vi "Execute Go Next Step.vi"(8 "error in (no error)":errorcluster, 11 "Chef Actor in":refnum<class "Chef Actor.lvclass">) -> (0 "error out":errorcluster, 3 "Chef Actor out":refnum<class "Chef Actor.lvclass">)   [LabVIEW 2024, in "Chef Actor.lvlib" / "Chef Actor.lvclass"]
uses:
  Chef Actor.lvclass
  Chef Actor.lvclass/Chef Actor.ctl
  Chef Actor Messages/Start Timer Msg/Start Timer Msg.lvclass
  Chef Actor Messages/Start Cooker Msg/Start Cooker Msg.lvclass
  <vilib>/ActorFramework/Actor/Actor.lvclass
  C:/Program Files/National Instruments/LabVIEW 2024/vi.lib/ActorFramework/Actor/Actor.lvclass
  G:/Leveling/LabVIEW/Learning/Actor Framework/chef/Chef Actor/Chef Actor.lvclass
  G:/Leveling/LabVIEW/Learning/Actor Framework/chef/Chef Actor Logic/Chef Actor Logic/Chef Actor Logic.lvclass
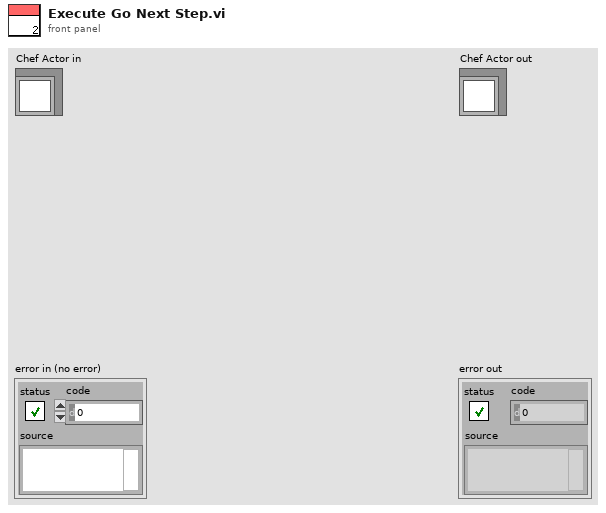
[diagram p1: front panel]
types:
  T1 = typedef "Step.ctl" = cluster{"Fire":dbl, "Duration":dbl}
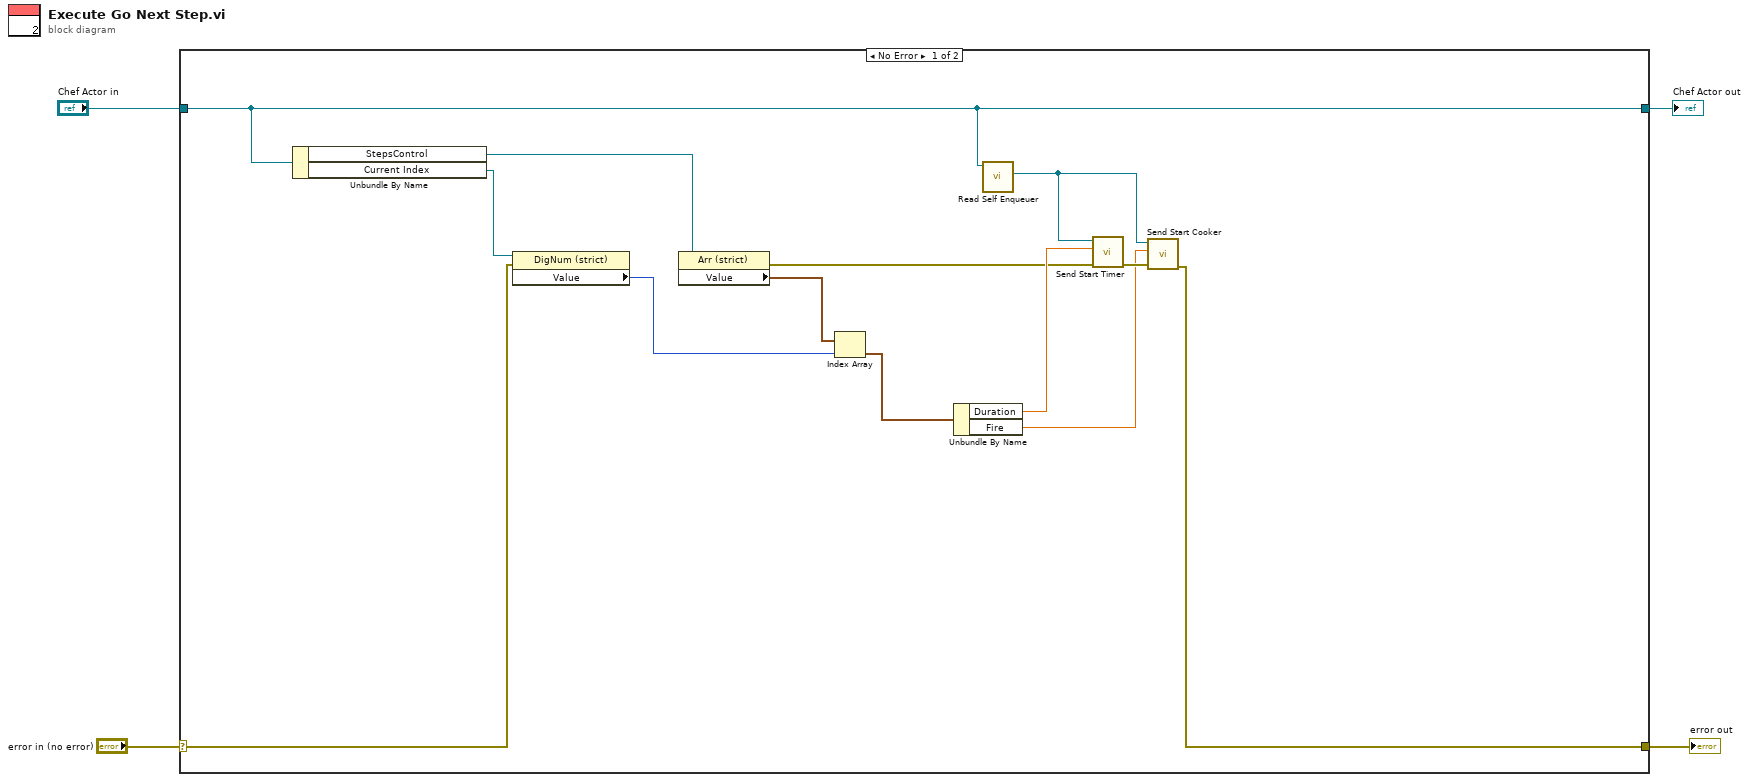
[diagram p0: block diagram]
diagram:
  n1 = case shown="No Error" "error in (no error)" {
    selector: "error in (no error)" -> [w6 w19]
    tunnel: [w5 w19] -> w3
    tunnel: [w11 w18] -> w1
    tunnel: "Chef Actor in" -> [w11 w18]
    frame No Error {
      n2 = Unbundle By Name(w11) -> ("StepsControl"=w17:refnum<vi>, "Current Index"=w16:refnum<vi>)
      n3 = property class="DigNum (strict)"(reference=w16, error in=w6) -> ("Value"=w14:i32)  [unwired: 2 out]
      n4 = property class="Arr (strict)"(reference=w17) -> (error out=w8:errorcluster, "Value"=w15:T1[])  [unwired: 1 in, 1 out]
      n5 = Index Array(array=w15, index=w14) -> (element=w12:T1)
      n6 = Unbundle By Name(w12) -> ("Duration"=w13:dbl, "Fire"=w7:dbl)
      n7 = call <vilib>:"Read Self Enqueuer.vi"("Actor"=w11) -> ("Self Enqueuer"=w10:refnum<class "Message Enqueuer.lvclass">)  [unwired: 10 in]
      n8 = call "Send Start Timer.vi"("error in (no error)"=w8, "Duration"=w13, "Message Enqueuer"=w10) -> ("error out"=w9:errorcluster)  [unwired: 7 in, 1 out]
      n9 = call "Send Start Cooker.vi"("error in (no error)"=w9, "Fire"=w7, "Message Enqueuer"=w10) -> ("error out"=w5:errorcluster)  [unwired: 7 in, 1 out]
    }
    frame Error {
    }
  }
  "error out" <- w3
  "Chef Actor out" <- w1
